vi "get update log.vi"(8 "error in (no error)":errorcluster, 11 "远端地址":string="/UP/OneStation/V4/版本升级文档.txt") -> (0 "error out":errorcluster, 2 "版本信息":cluster{"版本号":string, "更新内容":string}[](array[cluster]), 3 "元素":cluster{"版本号":string, "更新内容":string})   [LabVIEW 2016, in "数据传输系统-02.lvlib" / "update.lvlib"]
uses:
  update.lvlib
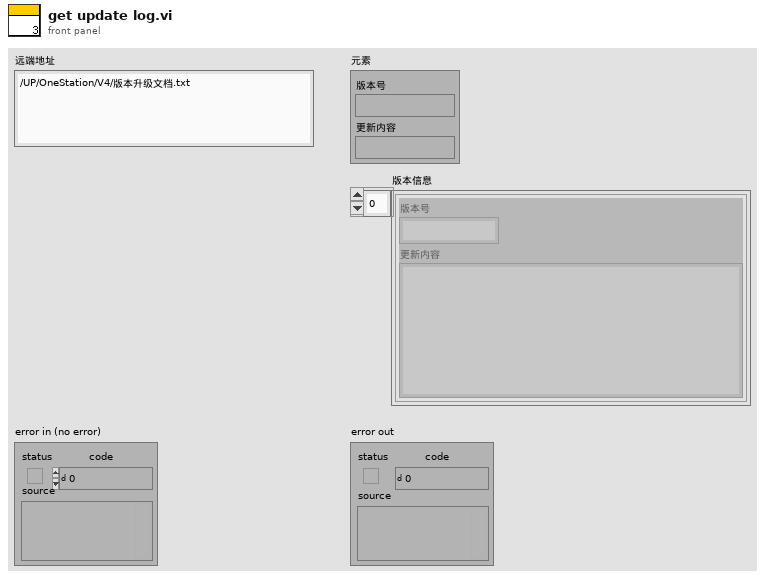
[diagram p1: front panel]
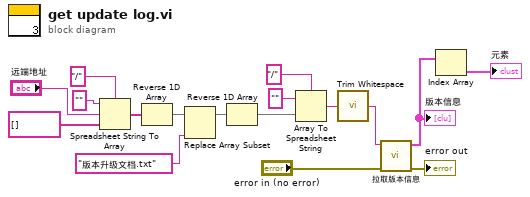
[diagram p0: block diagram]
diagram:
  n1 = Spreadsheet String To Array(delimiter (Tab)="/", format string="" ("格式字符串"), spreadsheet string="远端地址", array type (2D Dbl)=string[] []) -> (array=w10:string[])
  n2 = Reverse 1D Array(array=w10) -> (reversed array=w9:string[])
  n3 = Replace Array Subset(array=w9, new element="版本升级文档.txt") -> (w7:string[])  [unwired: 1 in]
  n4 = Reverse 1D Array(array=w7) -> (reversed array=w6:string[])
  n5 = Array To Spreadsheet String(delimiter (Tab)="/" ("分隔符(Tab)"), array=w6, 3:"" ("格式字符串")) -> (spreadsheet string=w3:string)
  n6 = call <vilib>:"Trim Whitespace.vi"("string"=w3) -> ("trimmed string"=w1:string)  [unwired: 1 in]
  n7 = call "拉取版本信息.vi"("error in (no error)"="error in (no error)", "远端地址"=w1) -> ("error out"=→"error out":errorcluster, "版本信息"=w17:cluster{"版本号":string, "更新内容":string}[])  [unwired: 8 in]
  "版本信息" <- w17
  n8 = Index Array(array=w17) -> (element=→"元素":cluster{"版本号":string, "更新内容":string})  [unwired: 1 in]
